vi "Close Handle.vi"(8 "error in (no error)":errorcluster, 11 "Handle":i64) -> (0 "error out":errorcluster, 3 "Sucess?":bool)   [LabVIEW 2018, in "Power Requests.lvlib"]
uses:
  Power Requests.lvlib
  kernel32.dll
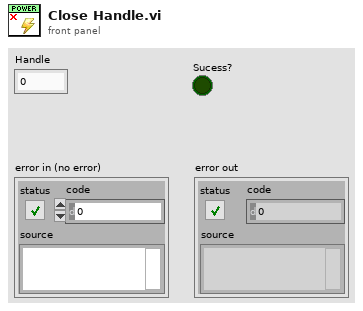
[diagram p1: front panel]
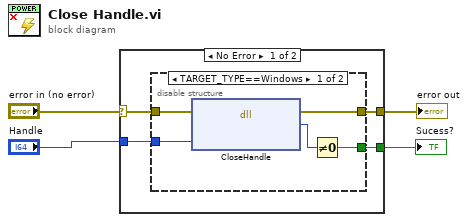
[diagram p0: block diagram]
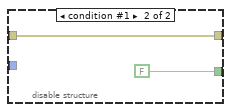
[diagram p2: hidden frame]
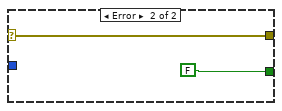
[diagram p3: hidden frame]
diagram:
  n1 = case shown="No Error" "error in (no error)" {
    selector: "error in (no error)" -> [w6 w17]
    tunnel: [w8 w17] -> w4
    tunnel: [w7 FALSE] -> w2
    tunnel: "Handle" -> [w5 _]
    frame No Error {
      n2 = disable-structure shown="TARGET_TYPE==Windows" {
        disable-tunnel: [w13 w15] -> w8
        disable-tunnel: [w12 FALSE] -> w7
        disable-tunnel: w6 -> [w11 w15]
        disable-tunnel: w5 -> [w9 _]
        frame condition #0 (active) {
          n3 = dll-call lib="kernel32.dll" fn="CloseHandle"(error in=w11, "_In_ HANDLE"=w9) -> (error out=w13:errorcluster, "BOOL"=w10:i32)  [unwired: 3 in, 1 out]
          n4 = Not Equal To 0?(x=w10) -> (x != 0?=w12:bool)
        }
        frame condition #1 {
        }
      }
    }
    frame Error {
    }
  }
  "error out" <- w4
  "Sucess?" <- w2
